vi "encodeStream.vi"(8 "error in (no error)":errorcluster, 11 "tBSONDocument in":refnum<class "tBSONDocument.lvclass">) -> (0 "error out":errorcluster, 2 "Byte Data":u8[](array[numeric]), 3 "tBSONDocument out":refnum<class "tBSONDocument.lvclass">)   [LabVIEW 2013, in "BSON.lvlib" / "tBSONDocument.lvclass"]
doc: "Generates the binary byte stream for this BSON document."
uses:
  tBSONDocument.lvclass
  tBSONDocument.lvclass/tBSONDocument.ctl
  tBSONElement/tBSONElement.lvclass
  BSON.lvlib
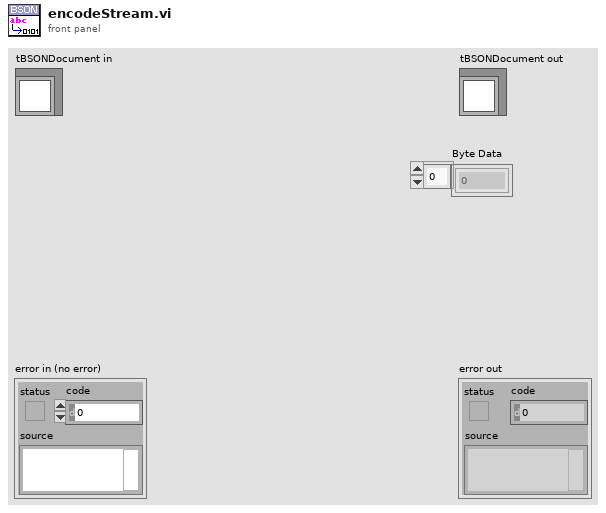
[diagram p1: front panel]
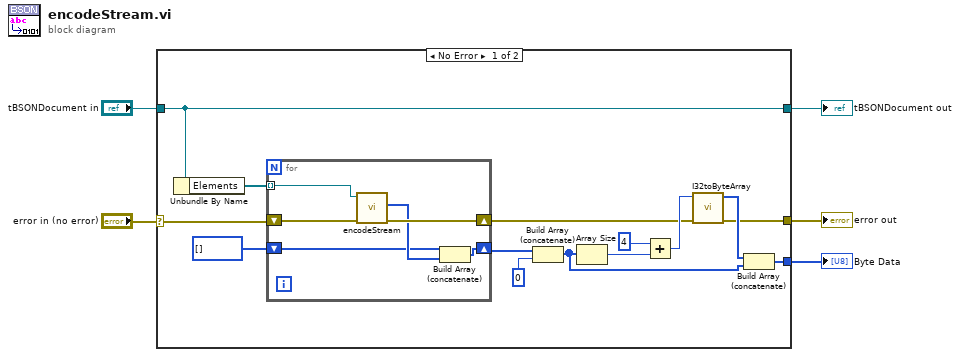
[diagram p0: block diagram]
diagram:
  n1 = case shown="No Error" "error in (no error)" {
    selector: "error in (no error)" -> [w18 w26]
    tunnel: [w19 w27] -> w3
    tunnel: "tBSONDocument in" -> [w19 w27]
    tunnel: [w10 w26] -> w2
    tunnel: [w9 _] -> w1
    frame No Error {
      n2 = Unbundle By Name(w19) -> ("Elements"=w7:refnum<class "tBSONElement.lvclass">[])
      n3 = for {
        shift-right: [w25] -> w17
        shift-left: u8[] [] -> [w22]
        tunnel: w7 -> [w20] mode=indexing
        shift-right: [w24] -> w6
        shift-left: w18 -> [w21]
        n4 = call-dynamic "encodeStream.vi"("error in (no error)"=w21, "tBSONElement in"=w20) -> ("error out"=w24:errorcluster, "Byte Array"=w23:u8[])  [unwired: 7 in, 1 out]
        n5 = Build Array (concatenate)(w22, w23) -> (w25:u8[])
      }
      n6 = Build Array (concatenate)(w17, u8 0) -> (w12:u8[])
      n7 = Array Size(array=w12) -> (size(s)=w15:i32)
      n8 = Add(x=4, y=w15) -> (x+y=w13:i32)
      n9 = call "I32toByteArray.vi"("error in (no error)"=w6, "I32"=w13) -> ("error out"=w10:errorcluster, "LittleEndianByteArray"=w11:u8[])  [unwired: 8 in]
      n10 = Build Array (concatenate)(w11, w12) -> (w9:u8[])
    }
    frame Error {
    }
  }
  "error out" <- w2
  "tBSONDocument out" <- w3
  "Byte Data" <- w1
